vi "Unpack for gRPC.vi"(8 "error in (no error)":errorcluster, 9 "Configuration / Resuls (Config)":enum16{"Configuration", "Results"}(ring), 10 "Any":T1, 11 "Measurement Customizations in":refnum<class "MeasurementPlugin.lvclass">) -> (0 "error out":errorcluster, 2 "Data Value":variant, 3 "Measurement Customizations out":refnum<class "MeasurementPlugin.lvclass">)   [LabVIEW 2021, in "Crosstalk_Class D Amplifier.lvlib" / "MeasurementPlugin.lvclass"]
uses:
  MeasurementPlugin.lvclass
  <vilib>/gRPC/LabVIEW gRPC Library/Shared/Any.ctl
  C:/Program Files/National Instruments/LabVIEW 2021/vi.lib/MeasurementLink/MeasurementLink Measurement Server/Measurement Plugin Service/Measurement Plugin Service.lvclass
  Measurement Configuration.ctl
  shared/controls/digital audio protocol/data justification.ctl
  shared/controls/digital audio protocol/endianness.ctl
  shared/controls/digital audio protocol/digital edge.ctl
  shared/controls/digital audio protocol/logic level.ctl
  shared/controls/digital output level units.ctl
  shared/controls/lowpass filter.ctl
  shared/controls/highpass filter.ctl
  Measurement Results.ctl
  a521b266-ce99-437c-923d-067dcf1e07fd.vi
  3ecd018e-d556-4cbc-bc60-c4ba57204520.vi
  <vilib>/gRPC/LabVIEW gRPC Library/Server API/Translate Protobuf Error.vi
  <vilib>/AdvancedString/1D String Array to Delimited String.vi
  <vilib>/gRPC/LabVIEW gRPC Library/Server API/Server/Get Server DLL Path.vi
  Crosstalk_Class D Amplifier.lvlib
  <vilib>/MeasurementLink/MeasurementLink Measurement Server/Measurement Plugin Service/Measurement Plugin Service.lvclass
  shared/controls/audio controls.lvlib
  <vilib>/gRPC/LabVIEW gRPC Library/grpc-lvsupport-release.lvlib
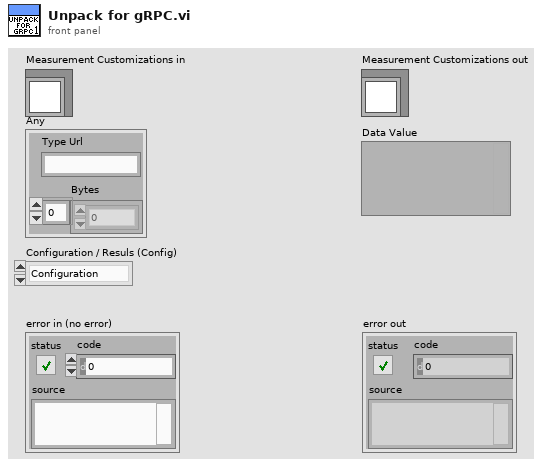
[diagram p1: front panel]
types:
  T1 = typedef "grpc-lvsupport-release.lvlib/Any.ctl" = cluster{"Type Url":string, "Bytes":u8[]}
  T2 = typedef "grpc-lvsupport-release.lvlib/grpcId.ctl" = u64
  T3 = typedef "Crosstalk_Class D Amplifier.lvlib/Measurement Configuration.ctl" = cluster{"digital channel list":string, "frame clock rate":dbl, "number of channels":u32, "channel length":u32, "bit depth":u32, "data justification":T4, "endianness":T5, "bit clock edge sync":T6, "frame sync edge for channel 0":T6, "channel 0 offset":u32, "master clock channel list":string, "master clock rate":dbl, "digital audio interferrer channel":i32, "logic level":T7, "signal frequency":dbl, "output level":dbl, "output level units":T8, "output range (pk-pk)":dbl, "load impedance":dbl, "signal phase":dbl, "acq sampling rate":dbl, "min measurement cycles":u32, "min measurement time (s)":dbl, "min settling cycles":u32, "min settling time (s)":dbl, "acq channel - victim":string, "acq channel - interferrer":string, "lowpass filter":T9, "highpass filter":T10}
  T4 = typedef "data justification.ctl" = enum32{"Left Justified", "Right Justified"}
  T5 = typedef "endianness.ctl" = enum32{"MSB First", "LSB First"}
  T6 = typedef "digital edge.ctl" = enum32{"Rising", "Falling"}
  T7 = typedef "logic level.ctl" = enum32{"3.3 V", "1.8 V", "1.2 V"}
  T8 = typedef "audio controls.lvlib/digital output level units.ctl" = enum32{"% FS", "dBFS"}
  T9 = typedef "lowpass filter.ctl" = enum32{"No filter", "AES17 20kHz", "AES17 40kHz"}
  T10 = typedef "highpass filter.ctl" = enum32{"DC", "AC"}
  T11 = typedef "Crosstalk_Class D Amplifier.lvlib/Measurement Results.ctl" = cluster{"channel name":string, "measured frequency (Hz)":dbl, "crosstalk (dB)":dbl, "output power (W)":dbl, "wfm - dt":dbl, "wfm_victim - data":dbl[], "wfm_interferrer - data":dbl[], "fft - f0":dbl, "fft - df":dbl, "fft_victim - data":dbl[], "fft_interferrer - data":dbl[]}
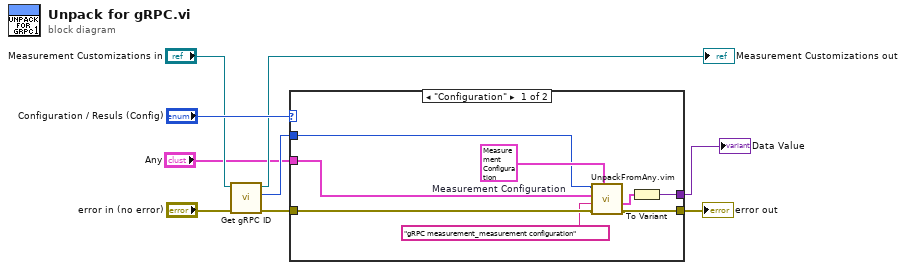
[diagram p0: block diagram]
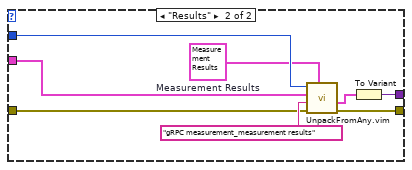
[diagram p2: hidden frame]
diagram:
  n1 = call <vilib>:"Get gRPC ID.vi"("error in"="error in (no error)", "measurement plugin service in"="Measurement Customizations in") -> ("error out"=w6:errorcluster, "gRPC ID"=w3:T2, "measurement plugin service out"=→"Measurement Customizations out":refnum<class "MeasurementPlugin.lvclass">)  [unwired: 7 in]
  n2 = case shown="\"Configuration\"" "Configuration / Resuls (Config)" {
    tunnel: w6 -> [w15 w19]
    tunnel: "Any" -> [w10 w18]
    tunnel: w3 -> [w12 w22]
    tunnel: [w16 w23] -> w9
    tunnel: [w17 w25] -> w1
    frame "Configuration" {
      w13 = T3 {"digital channel list"="7821\\PCMo 8", "frame clock rate"=48000.0, "number of channels"=2, "channel length"=32, "bit depth"=24, "data justification"=enum."Left Justified", "endianness"=enum."MSB First", "bit clock edge sync"=enum."Rising", "frame sync edge for channel 0"=enum."Rising", "channel 0 offset"=1, "master clock channel list"="7821\\PCMo 0", "master clock rate"=12288000.0, "digital audio interferrer channel"=0, "logic level"=enum."3.3 V", "signal frequency"=1000.0, "output level"=0.0, "output level units"=enum."% FS", "output range (pk-pk)"=3.16, "load impedance"=4.0, "signal phase"=0.0, "acq sampling rate"=1000.0, "min measurement cycles"=1000, "min measurement time (s)"=5.0, "min settling cycles"=0, "min settling time (s)"=0.0, "acq channel - victim"="", "acq channel - interferrer"="PXI1Slot4/ai0", "lowpass filter"=enum."No filter", "highpass filter"=enum."DC"}  # Measurement Configuration
      n3 = call "UnpackFromAny.vim"("Data Type"=w13, "error in"=w15, "Message Type"="gRPC measurement_measurement configuration", "Any"=w10, "gRPCid in"=w12) -> ("error out"=w16:errorcluster, "Unpacked Value"=w14:T3)  [unwired: 4 in, 1 out]
      n4 = To Variant(anything=w14) -> (Variant=w17:variant)
    }
    frame "Results" {
      w21 = T11 {"channel name"="", "measured frequency (Hz)"=0.0, "crosstalk (dB)"=0.0, "output power (W)"=0.0, "wfm - dt"=0.0, "wfm_victim - data"=[], "wfm_interferrer - data"=[], "fft - f0"=0.0, "fft - df"=0.0, "fft_victim - data"=[], "fft_interferrer - data"=[]}  # Measurement Results
      n5 = call "UnpackFromAny.vim"("Data Type"=w21, "error in"=w19, "Message Type"="gRPC measurement_measurement results", "Any"=w18, "gRPCid in"=w22) -> ("error out"=w23:errorcluster, "Unpacked Value"=w24:T11)  [unwired: 4 in, 1 out]
      n6 = To Variant(anything=w24) -> (Variant=w25:variant)
    }
  }
  "error out" <- w9
  "Data Value" <- w1
